vi "FTW-TestExecutive-Core_StepType_ConfigVI.vi"(0 "Step Actor":refnum<vi>, 1 "Other Config Items":string="{}", 5 "Inbox Address":string) -> (4 "Base Config String":string="{}")   [LabVIEW 2015, in "FTW-TestExecutive-Core.lvclass"]
uses:
  FTW-TestExecutive-Core.lvclass
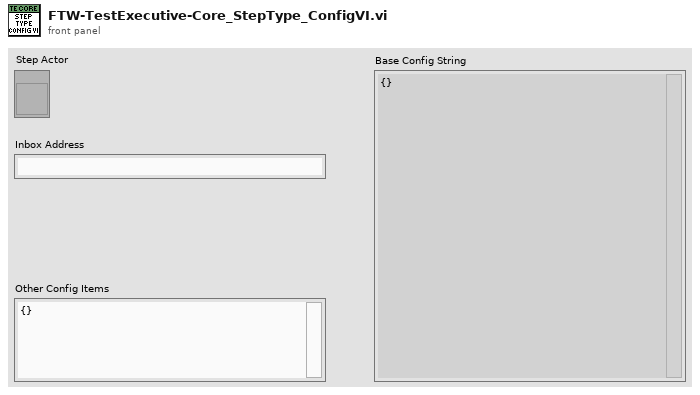
[diagram p1: front panel]
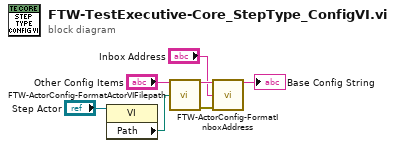
[diagram p0: block diagram]
diagram:
  n1 = property class="VI"(reference="Step Actor") -> ("Path"=w6:path)  [unwired: 1 in, 2 out]
  n2 = call "FTW-ActorConfig-FormatActorVIFilepath.vi"("FTW Config String In"="Other Config Items", "Actor VI Filepath"=w6) -> ("FTW Config String"=w4:string, "error out"=w3:errorcluster)  [unwired: 12 in]
  n3 = call "FTW-ActorConfig-FormatInboxAddress.vi"("FTW Config String In"=w4, "Inbox Address"="Inbox Address", "error in"=w3) -> ("FTW Config String"=→"Base Config String":string)  [unwired: 11 in, 1 out]
